vi "Version.vi"() -> (2 "Version":string)   [LabVIEW 2017]
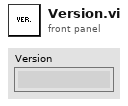
[diagram p1: front panel]
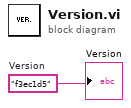
[diagram p0: block diagram]
diagram:
  w1 = "f3ec1d5"  # Version
  "Version" <- w1
